vi "Vision Calculations.vi"(0 "Image In":T2, 3 "error in":errorcluster) -> (5 "Vision Data":T1)   [LabVIEW 2013]
uses:
  <vilib>/vision/Image Controls.llb/IMAQ Image.ctl
  typedefs/Vision/vision data.ctl
  typedefs/Vision/vision enable.ctl
  <vilib>/vision/NI_Vision_Development_Module.lvlib
  typedefs/fg_typedef.ctl
panel:
  out "Aspect\nScore":dbl
  out "Rect Score":dbl
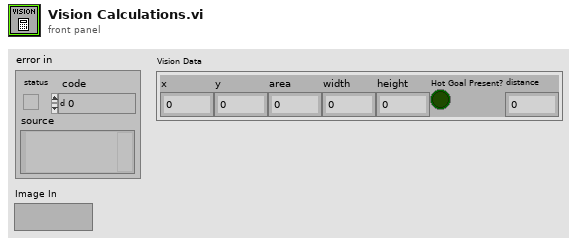
[diagram p1: front panel]
types:
  T1 = typedef "vision data.ctl" = cluster{"x":dbl, "y":dbl, "area":dbl, "width":dbl, "height":dbl, "Hot Goal Present?":bool, "distance":dbl}
  T2 = typedef "IMAQ Image.ctl" = refnum<image>
  T3 = typedef "Particle Parameters" = i32
  T4 = cluster{"Area":dbl, "Number of Holes":dbl, "Bounding Rect":cluster{"Left":dbl, "Top":dbl, "Right":dbl, "Bottom":dbl}, "Center of Mass":cluster{"X":dbl, "Y":dbl}, "Orientation":dbl, "Dimensions":cluster{"Width":dbl, "Height":dbl}}[]
  T5 = typedef "fg_typedef.ctl" = enum16{"Get", "Set"}
  T6 = typedef "vision enable.ctl" = enum16{"Enable", "Disable", "Stop"}
  T7 = cluster{"Horizontal":bool, "Aspect Score":dbl, "Rect Score":dbl, "Rectangle":cluster{"Left":dbl, "Top":dbl, "Right":dbl, "Bottom":dbl}, "Equiv H":dbl, "Equiv V":dbl}
  T8 = cluster{"Area":dbl, "Number of Holes":dbl, "Bounding Rect":cluster{"Left":dbl, "Top":dbl, "Right":dbl, "Bottom":dbl}, "Center of Mass":cluster{"X":dbl, "Y":dbl}, "Orientation":dbl, "Dimensions":cluster{"Width":dbl, "Height":dbl}}
  T9 = cluster{"Left":dbl, "Top":dbl, "Right":dbl, "Bottom":dbl}
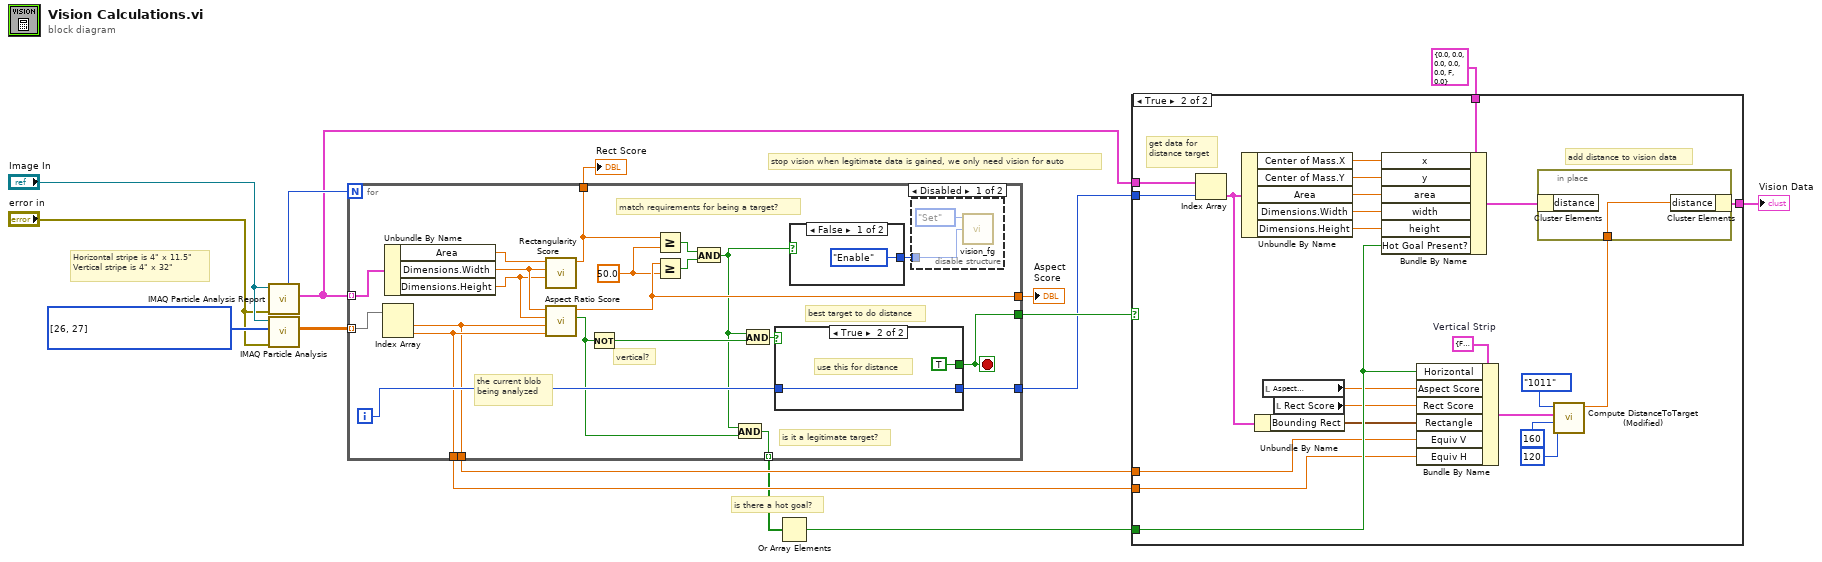
[diagram p0: block diagram]
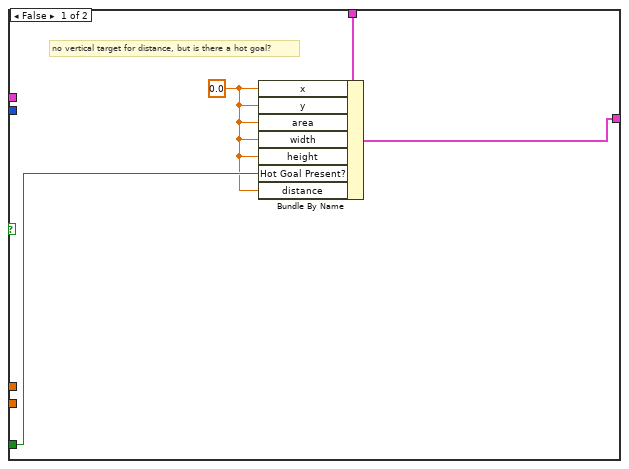
[diagram p2: hidden frame]
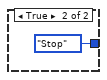
[diagram p4: hidden frame]
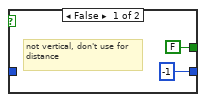
[diagram p5: hidden frame]
diagram:
  w14 = T3[] [26, 27] items=["Center of Mass X", "Center of Mass Y", "First Pixel X", "First Pixel Y", "Bounding Rect Left", "Bounding Rect Top", "Bounding Rect Right", "Bounding Rect Bottom", "Max Feret Diameter Start X", "Max Feret Diameter Start Y", "Max Feret Diameter End X", "Max Feret Diameter End Y", "Max Horiz. Segment Length Left", "Max Horiz. Segment Length Right", "Max Horiz. Segment Length Row", "-", "Bounding Rect Width", "Bounding Rect Height", "Bounding Rect Diagonal", "Perimeter", "Convex Hull Perimeter", "Holes' Perimeter", "Max Feret Diameter", "Equivalent Ellipse Major Axis", "Equivalent Ellipse Minor Axis", "Equivalent Ellipse Minor Axis (Feret)", "Equivalent Rect Long Side", "Equivalent Rect Short Side", "Equivalent Rect Diagonal", "Equivalent Rect Short Side (Feret)", "Average Horiz. Segment Length", "Average Vert. Segment Length", "Hydraulic Radius", "Waddel Disk Diameter", "-", "Area", "Holes' Area", "Particle & Holes' Area", "Convex Hull Area", "Image Area", "-", "Number of Holes", "Number of Horiz. Segments", "Number of Vert. Segments", "-", "Orientation", "Max Feret Diameter Orientation", "-", "% Area/Image Area", "% Area/(Particle & Holes' Area)", "Ratio of Equivalent Ellipse Axes", "Ratio of Equivalent Rect Sides", "-", "Elongation Factor", "Compactness Factor", "Heywood Circularity Factor", "Type Factor", "-", "Sum X", "Sum Y", "Sum XX", "Sum XY", "Sum YY", "Sum XXX", "Sum XXY", "Sum XYY", "Sum YYY", "-", "Moment of Inertia XX", "Moment of Inertia XY", "Moment of Inertia YY", "Moment of Inertia XXX", "Moment of Inertia XXY", "Moment of Inertia XYY", "Moment of Inertia YYY", "Norm. Moment of Inertia XX", "Norm. Moment of Inertia XY", "Norm. Moment of Inertia YY", "Norm. Moment of Inertia XXX", "Norm. Moment of Inertia XXY", "Norm. Moment of Inertia XYY", "Norm. Moment of Inertia YYY", "Hu Moment 1", "Hu Moment 2", "Hu Moment 3", "Hu Moment 4", "Hu Moment 5", "Hu Moment 6", "Hu Moment 7"] ("Pixel Measurements")
  # "stop vision when legitimate data is gained, we only need vision for auto"
  # "Horizontal stripe is 4\" x 11.5\"\nVertical stripe is 4\" x 32\""
  # "is there a hot goal?"
  n1 = call "IMAQ Particle Analysis Report"("error in (no error)"="error in", "Image"="Image In") -> ("Particle Reports (Pixels)"=w11:T4, "Number of Particles"=w16:i32)  [unwired: 4 in, 4 out]
  n2 = call "IMAQ Particle Analysis"("error in (no error)"="error in", "Pixel Measurements"=w14, "Image"="Image In") -> ("Particle Measurements (Pixels)"=w13:dbl[][])  [unwired: 3 in, 5 out]
  n3 = for {
    N: w16 -> [_]
    tunnel: w11 -> [w37] mode=indexing
    tunnel: w13 -> [w36] mode=indexing
    tunnel: [w29] -> w1
    tunnel: [w26] -> w9
    tunnel: [w25] -> w8
    tunnel: [w24] -> w6
    tunnel: [w23] -> w7
    tunnel: [w21] -> w3 mode=indexing
    tunnel: [w20] -> w2
    i -> [w28]
    stop <- w20 stop-if-true
    w17 = 50.0 ("aspect cutoff")
    # "is it a legitimate target?"
    # "the current blob\nbeing analyzed"
    # "match requirements for being a target?"
    # "best target to do distance"
    # "vertical?"
    n4 = Index Array(array=w36) -> (element #1=w23:dbl, element #2=w24:dbl)  [unwired: 2 in]
    n5 = Unbundle By Name(w37) -> ("Area"=w35:dbl, "Dimensions.Width"=w34:dbl, "Dimensions.Height"=w33:dbl)
    n6 = call "Rectangularity Score.vi"("Height"=w33, "Width"=w34, "Area"=w35) -> ("Score"=w26:dbl)  [unwired: 8 in]
    n7 = call "Aspect Ratio Score.vi"("Equivalent Rect Short"=w24, "Equivalent Rect Long"=w23, "Height"=w33, "Width"=w34) -> ("Horizontal"=w22:bool, "Score"=w25:dbl)  [unwired: 6 in]
    n8 = Not(x=w22) -> (.not. x?=w27:bool)
    n9 = Greater Or Equal?(x=w26, y=w17) -> (x >= y?=w31:bool)
    n10 = Greater Or Equal?(x=w25, y=w17) -> (x >= y?=w32:bool)
    n11 = And(x=w31, y=w32) -> (x .and. y?=w19:bool)
    n12 = And(x=w19, y=w22) -> (x .and. y?=w21:bool)
    n13 = And(x=w19, y=w27) -> (x .and. y?=w30:bool)
    n14 = case shown="True" w30 {
      tunnel: w28 -> [_ w45]
      tunnel: [-1 w45] -> w29
      tunnel: [FALSE TRUE] -> w20
      frame False {
        # "not vertical, don't use for\ndistance"
      }
      frame True {
        # "use this for distance"
      }
    }
    n15 = case shown="False" w19 {
      tunnel: [vision_enable."Enable" ("Action") vision_enable."Stop" ("Action")] -> w18
      frame False {
      }
      frame True {
      }
    }
    n16 = disable-structure shown="Disabled" {
      disable-tunnel: w18 -> [w38 _]
      frame Disabled {
        n17 = call "vision_fg.vi"("Action"=w38, "Menu"=fg_typedef."Set" ("Enum")) -> ()  [unwired: 1 in, 2 out]
      }
      frame Enabled {
      }
    }
  }
  "Rect Score" <- w9
  "Aspect\nScore" <- w8
  n18 = Or Array Elements(Boolean array=w3) -> (logical OR=w10:bool)
  n19 = case shown="True" w2 {
    tunnel: w11 -> [_ w72]
    tunnel: w10 -> [w47 w64]
    tunnel: w7 -> [_ w59]
    tunnel: w6 -> [_ w58]
    tunnel: [w48 w53] -> w5
    tunnel: w1 -> [_ w51]
    tunnel: T1 {"x"=0.0, "y"=0.0, "area"=0.0, "width"=0.0, "height"=0.0, "Hot Goal Present?"=FALSE, "distance"=0.0} ("Data") -> [w49 w50]
    frame False {
      w46 = 0.0
      # "no vertical target for distance, but is there a hot goal?"
      n20 = Bundle By Name(cluster=w49, "x"=w46, "y"=w46, "area"=w46, "width"=w46, "height"=w46, "Hot Goal Present?"=w47, "distance"=w46) -> (w48:T1)
    }
    frame True {
      w66 = T7 {"Horizontal"=FALSE, "Aspect Score"=0.0, "Rect Score"=0.0, "Rectangle"={"Left"=0.0, "Top"=0.0, "Right"=0.0, "Bottom"=0.0}, "Equiv H"=0.0, "Equiv V"=0.0}  # Vertical Strip
      # "add distance to vision data"
      # "get data for \ndistance target"
      n21 = Index Array(array=w72, index=w51) -> (element=w63:T8)
      n22 = Unbundle By Name(w63) -> ("Center of Mass.X"=w71:dbl, "Center of Mass.Y"=w70:dbl, "Area"=w69:dbl, "Dimensions.Width"=w68:dbl, "Dimensions.Height"=w67:dbl)
      n23 = Unbundle By Name(w63) -> ("Bounding Rect"=w62:T9)
      n24 = local read "Aspect\nScore"() -> (w60:dbl)
      n25 = local read "Rect Score"() -> (w61:dbl)
      n26 = Bundle By Name(cluster=w50, "x"=w71, "y"=w70, "area"=w69, "width"=w68, "height"=w67, "Hot Goal Present?"=w64) -> (w54:T1)
      n27 = Bundle By Name(cluster=w66, "Horizontal"=w64, "Aspect Score"=w60, "Rect Score"=w61, "Rectangle"=w62, "Equiv V"=w59, "Equiv H"=w58) -> (w65:T7)
      n28 = call "Compute DistanceToTarget (Modified).vi"("Y Image Resolution"=120, "X Image Resolution"=160, "Vertical Strip"=w65, "Camera Type"=enum16{"206", "1011", "1013"}."1011") -> ("Distance to Goal Wall (ft)"=w52:dbl)  [unwired: 5 in, 2 out]
      n29 = in-place {
        in-place-border: w52 -> [w73]
        n30 = in-place-cluster #1(w54) -> ()  [unwired: 1 out]
        n31 = in-place-cluster #1("distance"=w73) -> (w53:T1)
      }
    }
  }
  "Vision Data" <- w5
